vi "Init.vi"(5 "Scopes":string[](array[string]), 7 "Redirect URL (http://localhost)":refnum<class "URI.lvclass">, 10 "Token URL":refnum<class "URI.lvclass">, 11 "Auth URL":refnum<class "URI.lvclass">) -> (3 "Request out":refnum<class "Request.lvclass">)   [LabVIEW 2020, in "OAuth2.lvlib" / "Request.lvclass"]
uses:
  Request.lvclass
  Request.lvclass/Request.ctl
  <vilib>/IlluminatedG/lv-stream/URI/URI.lvclass
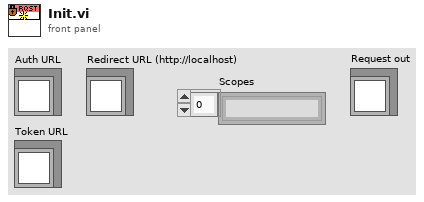
[diagram p1: front panel]
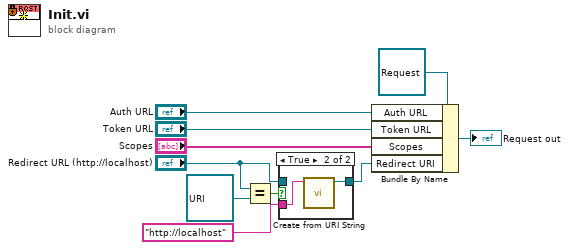
[diagram p0: block diagram]
diagram:
  n1 = Equal?(x="Redirect URL (http://localhost)", y=refnum<class "URI.lvclass"> refnum) -> (x = y?=w7:bool)
  n2 = case shown="True" w7 {
    tunnel: [w11 w12] -> w6
    tunnel: "http://localhost" -> [_ w13]
    tunnel: "Redirect URL (http://localhost)" -> [w11 _]
    frame False {
    }
    frame True {
      n3 = call <vilib>:"Create from URI String.vi"("URI String"=w13) -> ("URI out"=w12:refnum<class "URI.lvclass">)  [unwired: 9 in, 1 out]
    }
  }
  n4 = Bundle By Name(cluster=refnum<class "Request.lvclass"> refnum ("Request out"), "Auth URL"="Auth URL", "Token URL"="Token URL", "Scopes"="Scopes", "Redirect URI"=w6) -> (→"Request out":refnum<class "Request.lvclass">)
